vi "Get Point Iterator.vi"(0 "eye scan in":refnum<class "niHighSpeedSerial Rectangular Eye Scan v1 Host.lvclass">, 11 "error in":errorcluster) -> (4 "eye scan out":refnum<class "niHighSpeedSerial Rectangular Eye Scan v1 Host.lvclass">, 6 "eye scan point iterator":refnum<class "niHighSpeedSerial Eye Scan Point Iterator v1 Host.lvclass">, 15 "error out":errorcluster)   [LabVIEW 2014, in "niHighSpeedSerial Rectangular Eye Scan v1 Host.lvclass"]
doc: "Returns the Point Iterator.\n\n<B>Input Parameters</B>\n\n<B>eye scan in</B> Takes in a reference to your session from the previous VI.\n\n<B>error in</B> describes error conditions that occur before this node runs. This input provides standard 'error in' functionality.\n\n<B>Output Parameters</B>\n\n<B>eye scan out</B> passes a reference to your session to the next VI.\n\n<B>eye scan point iterator</B> is the incoming wire for the Eye Scan Point Iterator class object\n\n<B>error out</B> contains error information. This output provides standard 'error out' functionality."
uses:
  <instrlib>/niHighSpeedSerial/Eye Scan/v1/Host/Impl/Rectangular Eye Scan/niHighSpeedSerial Rectangular Eye Scan v1 Host.lvclass
  <instrlib>/niHighSpeedSerial/Eye Scan/v1/Host/Impl/Eye Scan Point Iterator/niHighSpeedSerial Eye Scan Point Iterator v1 Host.lvclass
  <instrlib>/niHighSpeedSerial/Eye Scan/v1/Host/Impl/Rectangular Eye Scan/niHighSpeedSerial Rectangular Eye Scan v1 Host.lvclass/niHighSpeedSerial Rectangular Eye Scan v1 Host.ctl
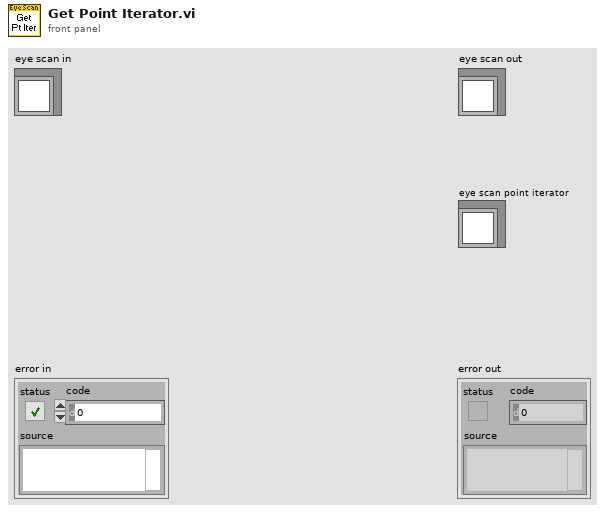
[diagram p1: front panel]
types:
  T1 = typedef "Rectangular Eye Scan v1 Host.lvclass/Private Data.ctl" = cluster{"horizontal step size":i16, "vertical step size":i16, "rectangular eye scan point iterator":refnum<class "niHighSpeedSerial Rectangular Eye Scan Point Iterator v1 Host.lvclass">}
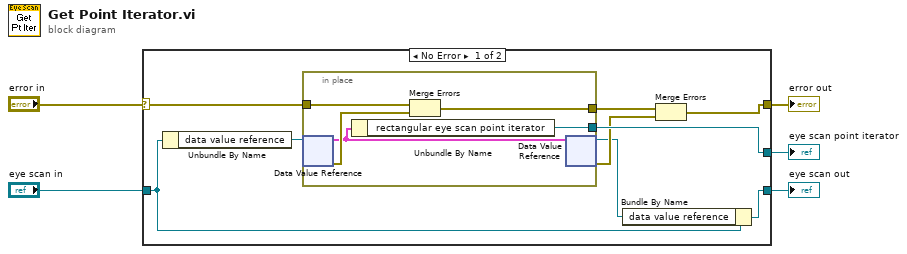
[diagram p0: block diagram]
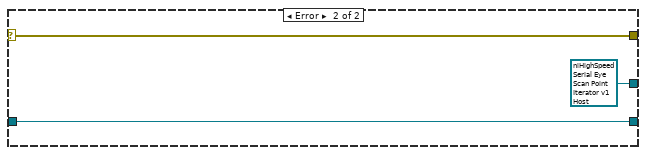
[diagram p2: hidden frame]
diagram:
  n1 = case shown="No Error" "error in" {
    selector: "error in" -> [w12 w22]
    tunnel: [w13 w22] -> w2
    tunnel: [w14 w21] -> w4
    tunnel: "eye scan in" -> [w11 w21]
    tunnel: [w9 refnum<class "niHighSpeedSerial Eye Scan Point Iterator v1 Host.lvclass"> refnum ("Point Iterator")] -> w1
    frame No Error {
      n2 = Unbundle By Name(w11) -> ("data value reference"=w10:refnum<data-value>)
      n3 = in-place {
        in-place-border: w12 -> [w19]
        in-place-border: [w17] -> w9
        in-place-border: [w16] -> w8
        n4 = in-place-dvr #1(w10) -> (w15:T1, w18:errorcluster)
        n5 = Unbundle By Name(w15) -> ("rectangular eye scan point iterator"=w17:refnum<class "niHighSpeedSerial Rectangular Eye Scan Point Iterator v1 Host.lvclass">)
        n6 = Merge Errors(w19, w18) -> (w16:errorcluster)
        n7 = in-place-dvr #1(w15) -> (w6:refnum<data-value>, w7:errorcluster)
      }
      n8 = Bundle By Name(cluster=w11, "data value reference"=w6) -> (w14:refnum<class "niHighSpeedSerial Rectangular Eye Scan v1 Host.lvclass">)
      n9 = Merge Errors(w8, w7) -> (w13:errorcluster)
    }
    frame Error {
    }
  }
  "error out" <- w2
  "eye scan out" <- w4
  "eye scan point iterator" <- w1
